vi "proceed.vi"(8 "error in (no error)":errorcluster, 11 "SweepDL090926Automation in":refnum<class "SweepDL090926Automation.lvclass">) -> (0 "error out":errorcluster, 3 "SweepDL090926Automation out":refnum<class "SweepDL090926Automation.lvclass">)   [LabVIEW 2010, in "SweepDL090926Automation.lvclass"]
uses:
  SweepDL090926Automation.lvclass
  common/clusters/plugin_specification.ctl
  SweepDL090926Automation.lvclass/SweepDL090926Automation.ctl
  ImagingMode/GenericImagingMode/GenericImagingMode/GenericImagingMode.lvclass
panel:
  out "current scan-mode specification":T1
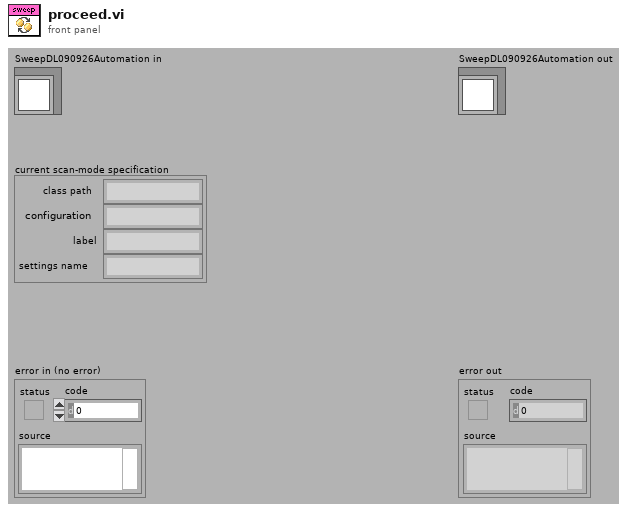
[diagram p1: front panel]
types:
  T1 = typedef "plugin_specification.ctl" = cluster{"class path":string, "configuration":string, "label":string, "settings name":string}
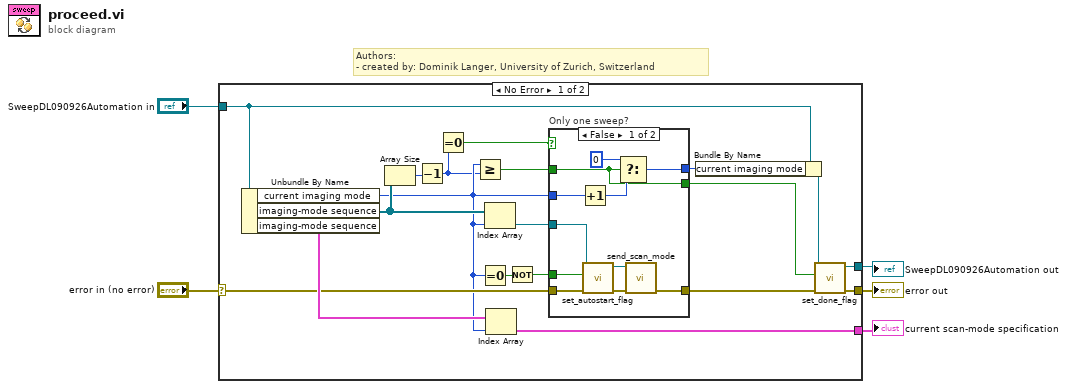
[diagram p0: block diagram]
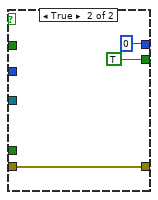
[diagram p2: hidden frame]
diagram:
  # "Authors: \n- created by: Dominik Langer, University of Zurich, Switzerland"
  n1 = case shown="No Error" "error in (no error)" {
    selector: "error in (no error)" -> [w18 w40]
    tunnel: [w15 w40] -> w4
    tunnel: "SweepDL090926Automation in" -> [w24 w39]
    tunnel: [w13 w39] -> w2
    tunnel: [w22 _] -> w1
    frame No Error {
      n2 = Unbundle By Name(w24) -> ("current imaging mode"=w17:i32, "imaging-mode sequence"=w21:refnum<class "GenericImagingMode.lvclass">[], "imaging-mode sequence"=w23:T1[])
      n3 = Array Size(array=w21) -> (size(s)=w19:i32)
      n4 = Decrement(x=w19) -> (x-1=w12:i32)
      n5 = Equal To 0?(x=w12) -> (x = 0?=w8:bool)
      n6 = Greater Or Equal?(x=w17, y=w12) -> (x >= y?=w7:bool)
      n7 = Equal To 0?(x=w17) -> (x = 0?=w10:bool)
      n8 = Index Array(array=w21, index=w17) -> (element=w11:refnum<class "GenericImagingMode.lvclass">)
      n9 = Index Array(array=w23, index=w17) -> (element=w22:T1)
      n10 = Not(x=w10) -> (.not. x?=w9:bool)
      n11 = case "Only one sweep?" shown="False" w8 {
        tunnel: [w35 0 ("t")] -> w20
        tunnel: w18 -> [w34 w38]
        tunnel: w17 -> [w33 _]
        tunnel: [w32 w38] -> w16
        tunnel: w7 -> [w25 _]
        tunnel: w11 -> [w27 _]
        tunnel: w9 -> [w26 _]
        tunnel: [w25 TRUE] -> w6
        frame False {
          n12 = Increment(x=w33) -> (x+1=w31:i32)
          n13 = call-dynamic "set_autostart_flag.vi"("error in (no error)"=w34, "autostart?"=w26, "GenericScanMode in"=w27) -> ("error out"=w29:errorcluster, "GenericScanMode out"=w28:refnum<class "GenericImagingMode.lvclass">)  [unwired: 7 in]
          n14 = Select(t=0, s=w25, f=w31) -> (s? t:f=w35:i32)
          n15 = call-dynamic "send_scan_mode.vi"("error in (no error)"=w29, "GenericScanMode in"=w28) -> ("error out"=w32:errorcluster)  [unwired: 8 in, 1 out]
        }
        frame True {
        }
      }
      n16 = Bundle By Name(cluster=w24, "current imaging mode"=w20) -> (w14:refnum<class "SweepDL090926Automation.lvclass">)
      n17 = call-dynamic "set_done_flag.vi"("error in (no error)"=w16, "done?"=w6, "GenericSweep in"=w14) -> ("error out"=w15:errorcluster, "GenericSweep out"=w13:refnum<class "SweepDL090926Automation.lvclass">)  [unwired: 7 in]
    }
    frame Error {
    }
  }
  "error out" <- w4
  "SweepDL090926Automation out" <- w2
  "current scan-mode specification" <- w1
